vi "Read.vi"(8 "error in (no error)":errorcluster, 11 "Numeric in":refnum<class "Var_Variant.lvclass">) -> (0 "error out":errorcluster, 2 "Value":T1=variant(string ""), 3 "Numeric out":refnum<class "Var_Variant.lvclass">)   [LabVIEW 2021, in "Var_Variant.lvclass"]
uses:
  Var_Variant.lvclass
  Type.ctl
  Var_Variant.lvclass/Var_Variant.ctl
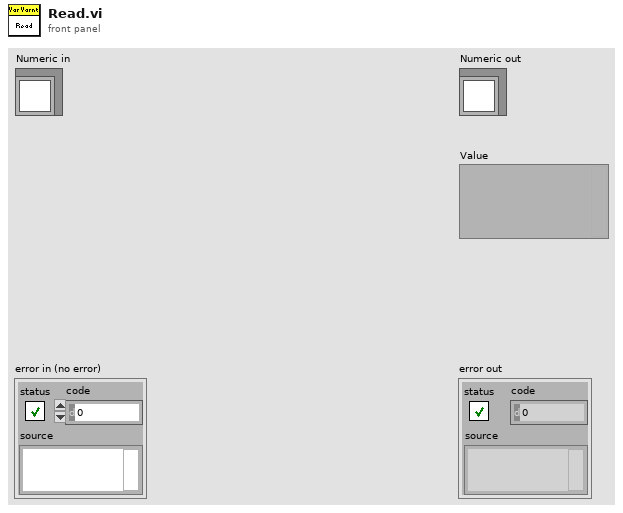
[diagram p1: front panel]
types:
  T1 = typedef "Var_Variant.lvclass/Type.ctl" = variant
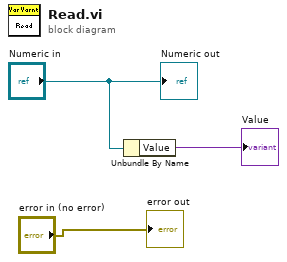
[diagram p0: block diagram]
diagram:
  n1 = Unbundle By Name("Numeric in") -> ("Value"=→"Value":T1)
  "error out" <- "error in (no error)"
  "Numeric out" <- "Numeric in"
